vi "Show Hide Cursor.vi"(0 "State":T1) -> ()   [LabVIEW 2020, in "Interactive Graph.xctl"]
uses:
  Interactive Graph.xctl
  State.vi
  Persistent.ctl
  Plot.ctl
  Label Position.ctl
  Events.ctl
  Selection.ctl
  XRange.ctl
  YScale.ctl
  Cursor.ctl
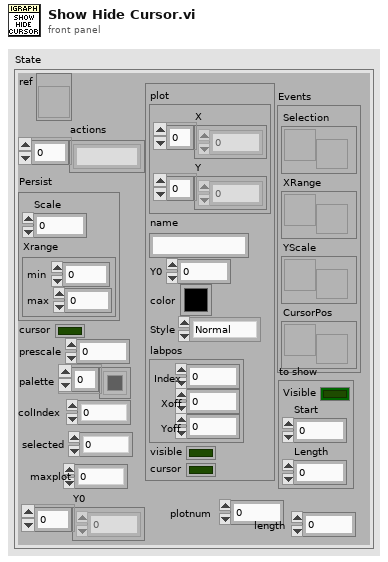
[diagram p1: front panel]
types:
  T1 = typedef "Interactive Graph.xctl/State.vi" = cluster{"ref":refnum<vi>, "actions":string[], "Persist":T2, "cursor":bool, "prescale":dbl, "palette":u32[], "colIndex":i32, "to add":T3, "Events":T5, "selected":i32, "to show":cluster{"Visible":bool, "Start":i32, "Length":i32}, "maxplot":i32, "Y0":dbl[], "plotnum":i32, "length":i32}
  T2 = typedef "Interactive Graph.xctl/Persistent.ctl" = cluster{"Scale":dbl, "Xrange":cluster{"min":dbl, "max":dbl}}
  T3 = typedef "Interactive Graph.xctl/Plot.ctl" = cluster{"plot":cluster{"X":dbl[], "Y":dbl[]}, "name":string, "Y0":dbl, "color":u32, "Style":enum16{"Normal", "Highlight", "Shadow"}, "labpos":T4, "visible":bool, "cursor":bool}
  T4 = typedef "Label Position.ctl" = cluster{"Index":i32, "Xoff":dbl, "Yoff":dbl}
  T5 = typedef "Interactive Graph.xctl/Events.ctl" = cluster{"Selection":refnum<user-event>, "XRange":refnum<user-event>, "YScale":refnum<user-event>, "CursorPos":refnum<user-event>}
  T6 = typedef "LVCursorListTypeDef.ctl" = cluster{"Name":string, "Color":u32, "Style":u8, "Point Style":u8, "Name Visible":bool, "Allow Drag":bool, "Cursor Mode":u32, "Plot":i32, "Index":i32, "Position":cluster{"X":dbl, "Y":dbl}, "X Scale":u32, "Y Scale":u32, "Watch Plots":i32[], "Watch All Plots":bool, "Plot Area":i32, "Label Offset":cluster{"X":dbl, "Y":dbl}}[]
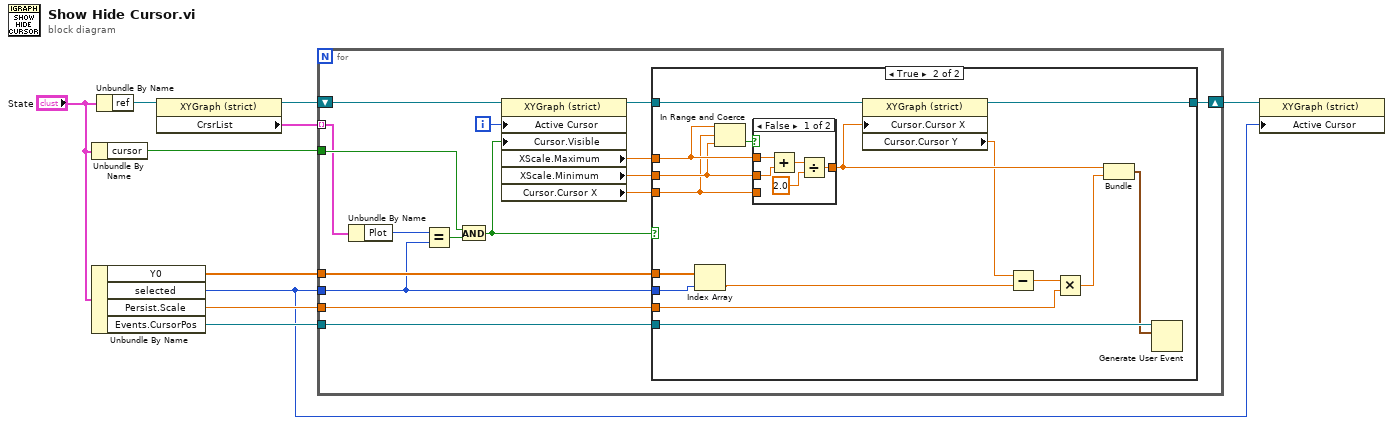
[diagram p0: block diagram]
diagram:
  n1 = Unbundle By Name("State") -> ("cursor"=w7:bool)
  n2 = Unbundle By Name("State") -> ("Y0"=w3:dbl[], "selected"=w1:i32, "Persist.Scale"=w4:dbl, "Events.CursorPos"=w5:refnum<user-event>)
  n3 = Unbundle By Name("State") -> ("ref"=w10:refnum<vi>)
  n4 = property class="XYGraph (strict)"(reference=w10) -> (reference out=w8:refnum<vi>, "CrsrList"=w9:T6)  [unwired: 1 in, 1 out]
  n5 = for {
    tunnel: w9 -> [w13] mode=indexing
    shift-right: [w20] -> w2
    shift-left: w8 -> [w26]
    tunnel: w7 -> [w23]
    tunnel: w5 -> [w16]
    tunnel: w3 -> [w15]
    tunnel: w4 -> [w14]
    tunnel: w1 -> [w11]
    i -> [w25]
    n6 = Unbundle By Name(w13) -> ("Plot"=w12:i32)
    n7 = Equal?(x=w12, y=w11) -> (x = y?=w24:bool)
    n8 = And(x=w23, y=w24) -> (x .and. y?=w22:bool)
    n9 = property class="XYGraph (strict)"(reference=w26, "Active Cursor"=w25, "Cursor.Visible"=w22) -> (reference out=w21:refnum<vi>, "XScale.Maximum"=w19:dbl, "XScale.Minimum"=w18:dbl, "Cursor.Cursor X"=w17:dbl)  [unwired: 1 in, 1 out]
    n10 = case shown="True" w22 {
      tunnel: w21 -> [w27 w43]
      tunnel: [w27 w42] -> w20
      tunnel: w19 -> [_ w40]
      tunnel: w18 -> [_ w39]
      tunnel: w17 -> [_ w38]
      tunnel: w16 -> [_ w36]
      tunnel: w15 -> [_ w34]
      tunnel: w14 -> [_ w29]
      tunnel: w11 -> [_ w28]
      frame False {
      }
      frame True {
        n11 = Index Array(array=w34, index=w28) -> (element=w32:dbl)
        n12 = In Range and Coerce(upper limit=w40, x=w38, lower limit=w39) -> (In Range?=w41:bool)  [unwired: 1 out]
        n13 = case shown="False" w41 {
          tunnel: w38 -> [_ w49]
          tunnel: [w44 w49] -> w37
          tunnel: w39 -> [w48 _]
          tunnel: w40 -> [w47 _]
          frame False {
            n14 = Add(x=w47, y=w48) -> (x+y=w46:dbl)
            n15 = Divide(x=w46, y=2.0) -> (x/y=w44:dbl)
          }
          frame True {
          }
        }
        n16 = property class="XYGraph (strict)"(reference=w43, "Cursor.Cursor X"=w37) -> (reference out=w42:refnum<vi>, "Cursor.Cursor Y"=w30:dbl)  [unwired: 1 in, 1 out]
        n17 = Subtract(x=w30, y=w32) -> (x-y=w33:dbl)
        n18 = Multiply(x=w33, y=w29) -> (x*y=w31:dbl)
        n19 = Bundle("Cursor.Cursor X"=w37, w31) -> (w35:cluster{"Cursor.Cursor X":dbl, dbl})  [unwired: 1 in]
        n20 = Generate User Event(user event=w36, event data cluster=w35) -> ()  [unwired: 2 in, 2 out]
      }
    }
  }
  n21 = property class="XYGraph (strict)"(reference=w2, "Active Cursor"=w1) -> ()  [unwired: 1 in, 2 out]
